vi "excecuteCommand.vi"(8 "error in (no error)":errorcluster, 9 "input":variant, 10 "MonoCommand":T1=enum."getStatus", 11 "MonoClientCommunicator in":refnum<class "MonoClientCommunicator.lvclass">) -> (0 "error out":errorcluster, 1 "parameter":T2, 2 "value":variant, 3 "MonoClientCommunicator out":refnum<class "MonoClientCommunicator.lvclass">)   [LabVIEW 2016, in "MonoClientCommunicator.lvclass"]
uses:
  MonoClientCommunicator.lvclass
  Typedefs/publishers.ctl
  Typedefs/MonoCommand.ctl
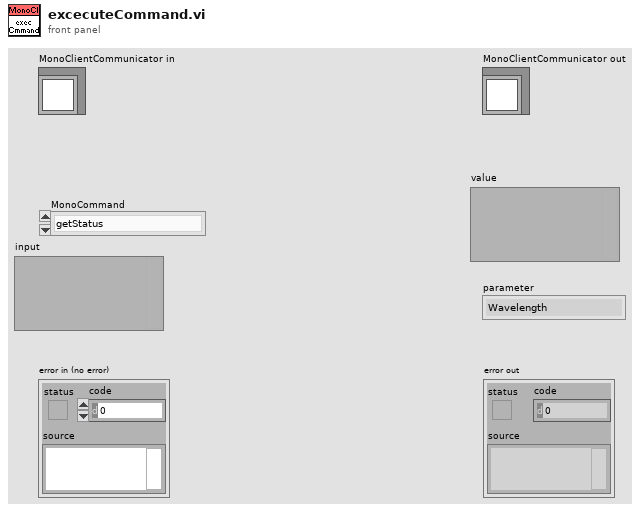
[diagram p1: front panel]
types:
  T1 = typedef "MonoCommand.ctl" = enum16{"getGrating", "getFrontEntranceSlitPosition", "getFrontExitSlitPosition", "getWavelength", "setWavelength", "setGrating", "setFrontEntranceSlitPosition", "setFrontExitSlitPosition", "calibrateWavelength", "getStatus", "Unknown", "reset", "setAll"}
  T2 = typedef "publishers.ctl" = enum16{"Wavelength", "Grating", "FrontEntranceSlitPosition", "FrontExitSlitPosition", "SoftwareStatus", "MonochromatorId", "Ack"}
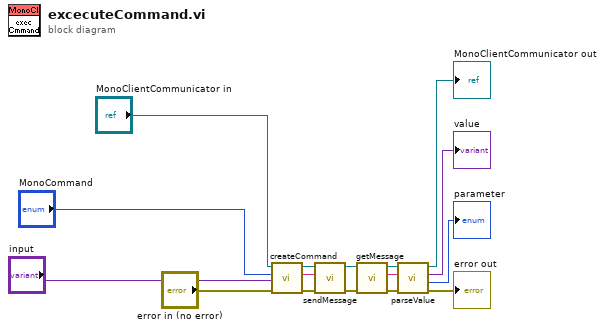
[diagram p0: block diagram]
diagram:
  n1 = call "createCommand.vi"("error in (no error)"="error in (no error)", "Variant"="input", "MonoCommand"="MonoCommand", "MonoClientCommunicator in"="MonoClientCommunicator in") -> ("error out"=w9:errorcluster, "command"=w10:string, "MonoClientCommunicator out"=w11:refnum<class "MonoClientCommunicator.lvclass">)  [unwired: 5 in]
  n2 = call "sendMessage.vi"("error in (no error)"=w9, "message"=w10, "MonoClientCommunicator in"=w11) -> ("error out"=w12:errorcluster, "MonoClientCommunicator out"=w13:refnum<class "MonoClientCommunicator.lvclass">)  [unwired: 7 in]
  n3 = call "getMessage.vi"("error in (no error)"=w12, "MonoClientCommunicator in"=w13) -> ("error out"=w15:errorcluster, "message"=w16:string, "MonoClientCommunicator out"=w14:refnum<class "MonoClientCommunicator.lvclass">)  [unwired: 7 in]
  n4 = call "parseValue.vi"("error in (no error)"=w15, "message"=w16, "MonoClientCommunicator in"=w14) -> ("error out"=→"error out":errorcluster, "parameter"=→"parameter":T2, "value"=→"value":variant, "MonoClientCommunicator out"=→"MonoClientCommunicator out":refnum<class "MonoClientCommunicator.lvclass">)  [unwired: 5 in]
